vi "FPGA FK.vi"() -> ()   [LabVIEW 2015]
uses:
  <vilib>/rvi/FXPMathLib/FxpSinAndCos/subVIs/nifxpmath_SinAndCos_SimConfig.ctl
  <vilib>/rvi/Emulation/niFpgaGetClockAttributes.vi
  <vilib>/rvi/Emulation/niFpgaSctlEmulationGetInTimedLoop.vi
  <vilib>/rvi/Emulation/niFpgaEmulationReportErrorSimple.vi
  <vilib>/rvi/FXPMathLib/FxpSinAndCos/simVIs/DllFxpSinAndCosTemp_sub.vi
  <vilib>/rvi/Emulation/niFpgaCriticalErrorInLSC.vi
  <vilib>/rvi/FXPMathLib/FxpSinAndCos/XNode/nifxpmath_SinAndCos.xnode
panel:
  in  "LINK2_ENC_POS":i32
  in  "LINK1_ENC_POS":i32=-9000
  in  "LINK1_LENGTH_MM":fxp<+,16,12>=345.0 format="%#_19g"
  in  "LINK2_LENGTH_MM":fxp<+,16,12>=235.0 format="%#_19g"
  out "LINK1_X_MM":fxp<+/-,34,16>=-123.92059326171875
  out "LINK1_Y_MM":fxp<+/-,34,16>=686.492919921875
  in  "X_OFFSET_MM":fxp<+/-,33,15>=-200.0
  in  "Y_OFFSET_MM":fxp<+/-,33,15>=350.0
  out "LINK2_Y_MM":fxp<+/-,34,16>=915.6982421875
  out "LINK2_X_MM":fxp<+/-,34,16>=-72.098388671875
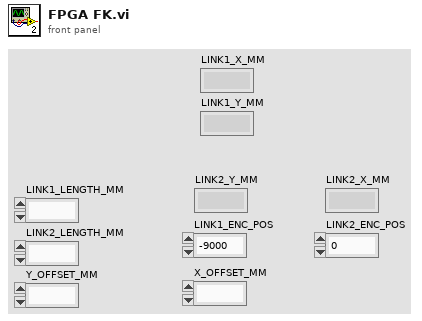
[diagram p1: front panel]
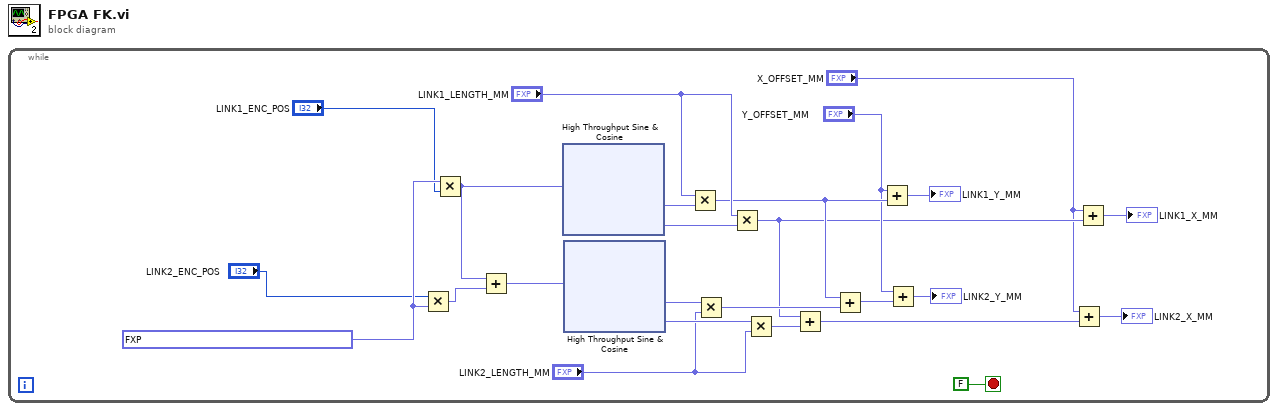
[diagram p0: block diagram]
diagram:
  n1 = while {
    stop <- FALSE stop-if-true
    w4 = fxp<+,31,-8> 5.555555617320351e-05
    n2 = Multiply(x="LINK2_ENC_POS", y=w4) -> (x*y=w24:fxp<+/-,63,24>)
    n3 = Multiply(x=w4, y="LINK1_ENC_POS") -> (x*y=w3:fxp<+/-,63,24>)
    n4 = Add(x=w3, y=w24) -> (x+y=w23:fxp<+/-,64,25>)
    n5 = xnode "High Throughput Sine & Cosine"("x (pi)"=w3) -> ("sin(x)"=w22:fxp<+/-,16,2>, "cos(x)"=w21:fxp<+/-,16,2>)
    n6 = xnode "High Throughput Sine & Cosine"("x (pi)"=w23) -> ("sin(x)"=w19:fxp<+/-,16,2>, "cos(x)"=w18:fxp<+/-,16,2>)
    n7 = Multiply(x="LINK1_LENGTH_MM", y=w22) -> (x*y=w14:fxp<+/-,32,14>)
    n8 = Multiply(x=w19, y="LINK2_LENGTH_MM") -> (x*y=w15:fxp<+/-,32,14>)
    n9 = Multiply(x="LINK1_LENGTH_MM", y=w21) -> (x*y=w9:fxp<+/-,32,14>)
    n10 = Multiply(x=w18, y="LINK2_LENGTH_MM") -> (x*y=w16:fxp<+/-,32,14>)
    n11 = Add(x=w9, y=w16) -> (x+y=w7:fxp<+/-,33,15>)
    n12 = Add(x=w14, y=w15) -> (x+y=w13:fxp<+/-,33,15>)
    n13 = Add(x="Y_OFFSET_MM", y=w14) -> (x+y=→"LINK1_Y_MM":fxp<+/-,34,16>)
    n14 = Add(x="Y_OFFSET_MM", y=w13) -> (x+y=→"LINK2_Y_MM":fxp<+/-,34,16>)
    n15 = Add(x="X_OFFSET_MM", y=w7) -> (x+y=→"LINK2_X_MM":fxp<+/-,34,16>)
    n16 = Add(x="X_OFFSET_MM", y=w9) -> (x+y=→"LINK1_X_MM":fxp<+/-,34,16>)
  }
